vi "Configure Trigger (TV).vi"(0 "VISA resource name":refnum<visa-resource-name>, 1 "Signal Format (0: NTSC)":u16(ring) items=["NTSC", "PAL", "User Defined"], 2 "Event (1: Field 1)":u16(ring)=1 items=[" Field 1"=1, " Field 2"=2], 3 "Line Number (1)":i32=1, 5 "Trigger Source (1: Channel 1)":u16(ring)=1 items=["Channel 1"=1, "Channel 2"=2, "Channel 3"=3, "Channel 4"=4], 7 "Trigger Level (0.0 V)":dbl, 9 "Trigger Polarity (0: Positive)":u16(ring) items=["Positive", "Negative"], 11 "error in (no error)":errorcluster, 12 "UDTV Min Width (26e-6)":dbl=2.6e-05, 13 "UDTV Edge Number (1)":i32=1) -> (4 "VISA resource name out":refnum<visa-resource-name>, 15 "error out":errorcluster)   [LabVIEW 2012, in "Agilent 8000 Series.lvlib"]
doc: "Configures the TV trigger. You configure the TV trigger source, signal format, the event on which to trigger, the signal polarity and other polarities."
uses:
  Agilent 8000 Series.lvlib
panel:
  # "NTSC or PAL"
  # "User Defined Format"
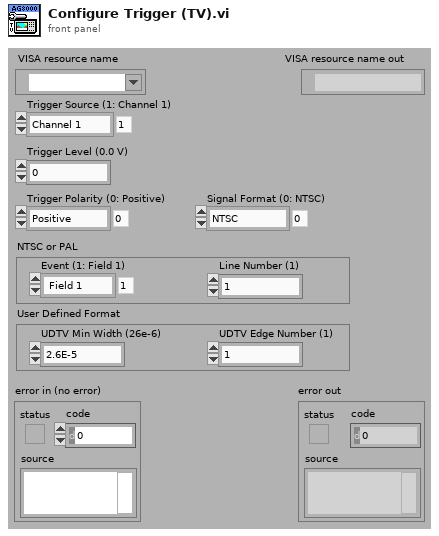
[diagram p1: front panel]
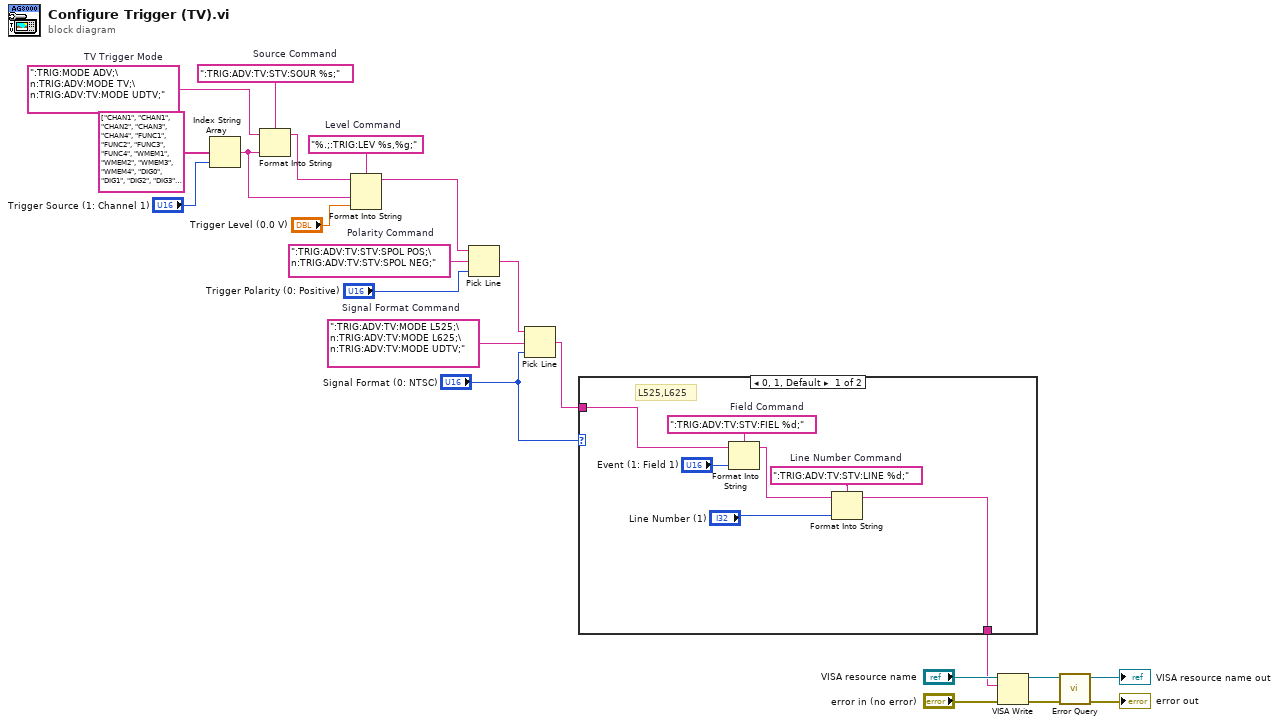
[diagram p0: block diagram]
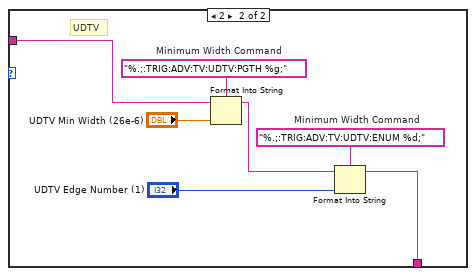
[diagram p2: hidden frame]
diagram:
  w5 = ":TRIG:ADV:TV:MODE L525;\n:TRIG:ADV:TV:MODE L625;\n:TRIG:ADV:TV:MODE UDTV;"  # Signal Format Command
  w8 = "%.;:TRIG:LEV %s,%g;"  # Level Command
  w12 = ":TRIG:ADV:TV:STV:SPOL POS;\n:TRIG:ADV:TV:STV:SPOL NEG;"  # Polarity Command
  w13 = ":TRIG:ADV:TV:STV:SOUR %s;"  # Source Command
  w14 = ":TRIG:MODE ADV;\n:TRIG:ADV:MODE TV;\n:TRIG:ADV:TV:MODE UDTV;"  # TV Trigger Mode
  n1 = Index String Array(1:"Trigger Source (1: Channel 1)", 2:string[] ["CHAN1", "CHAN1", "CHAN2", "CHAN3", "CHAN4", "FUNC1", "FUNC2", "FUNC3", "FUNC4", "WMEM1", "WMEM2", "WMEM3", "WMEM4", "DIG0", "DIG1", "DIG2", "DIG3", "DIG4", "DIG5", "DIG6", "DIG7", "DIG8", "DIG9", "DIG10", "DIG11", "DIG12", "DIG13", "DIG14", "DIG15", "AUX", "LINE"]) -> (0:w10:string)  [unwired: 1 in]
  n2 = Format Into String(format string=w13, initial string=w14, w10) -> (resulting string=w7:string)  [unwired: 1 in, 1 out]
  n3 = Format Into String(format string=w8, initial string=w7, w10, "Trigger Level (0.0 V)") -> (resulting string=w6:string)  [unwired: 1 in, 1 out]
  n4 = Pick Line(string ("")=w6, multi-line string=w12, line index="Trigger Polarity (0: Positive)") -> (output string=w4:string)
  n5 = Pick Line(string ("")=w4, multi-line string=w5, line index="Signal Format (0: NTSC)") -> (output string=w2:string)
  n6 = case shown="0, 1, Default" "Signal Format (0: NTSC)" {
    tunnel: w2 -> [w29 w34]
    tunnel: [w23 w30] -> w1
    frame 0, 1, Default {
      w25 = ":TRIG:ADV:TV:STV:LINE %d;"  # Line Number Command
      w27 = ":TRIG:ADV:TV:STV:FIEL %d;"  # Field Command
      # "L525,L625"
      n7 = Format Into String(format string=w27, initial string=w29, "Event (1: Field 1)") -> (resulting string=w24:string)  [unwired: 1 in, 1 out]
      n8 = Format Into String(format string=w25, initial string=w24, "Line Number (1)") -> (resulting string=w23:string)  [unwired: 1 in, 1 out]
    }
    frame 2 {
      w33 = "%.;:TRIG:ADV:TV:UDTV:ENUM %d;"  # Minimum Width Command
      w36 = "%.;:TRIG:ADV:TV:UDTV:PGTH %g;"  # Minimum Width Command
      # "UDTV"
      n9 = Format Into String(format string=w36, initial string=w34, "UDTV Min Width (26e-6)") -> (resulting string=w32:string)  [unwired: 1 in, 1 out]
      n10 = Format Into String(format string=w33, initial string=w32, "UDTV Edge Number (1)") -> (resulting string=w30:string)  [unwired: 1 in, 1 out]
    }
  }
  n11 = VISA Write(VISA resource name="VISA resource name", write buffer=w1, error in (no error)="error in (no error)") -> (VISA resource name out=w18:refnum<visa-resource-name>, error out=w17:errorcluster)  [unwired: 1 out]
  n12 = call "Error Query.vi"("error in (no error)"=w17, "VISA resource name"=w18) -> ("error out"=→"error out":errorcluster, "VISA resource name out"=→"VISA resource name out":refnum<visa-resource-name>)  [unwired: 6 in, 2 out]
